vi "TCL Get Signal.vi"(3 "event number":i32, 4 "error in (no error)":errorcluster, 5 "signal name":string, 7 "event file":path) -> (0 "error out":errorcluster, 1 "signal":dbl[](array[numeric]))   [LabVIEW 2010]
doc: "This VI looks up the requested event number and then compares its rf frequency and modulation with the input values. If the event is found, and if the frequency and modulation match, the raw signal of the baseline is returned. Otherwise, an empty array is returned."
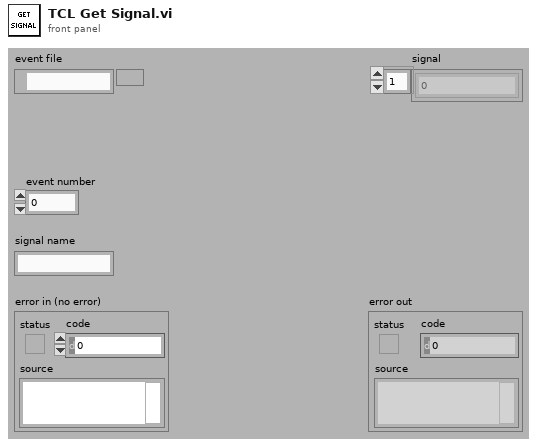
[diagram p1: front panel]
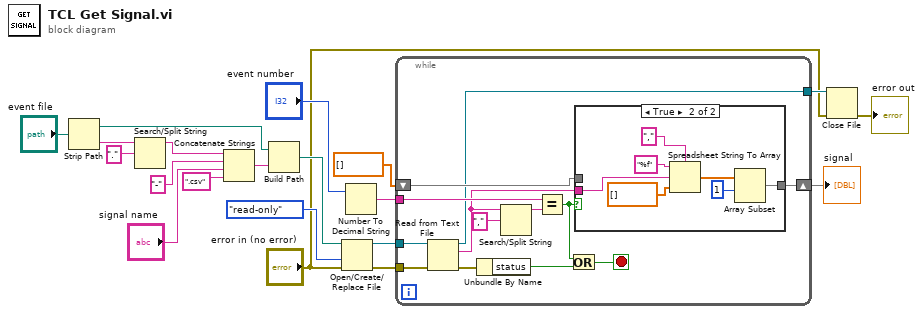
[diagram p0: block diagram]
diagram:
  n1 = Strip Path(path="event file") -> (stripped path=w4:path, name=w3:string)
  n2 = Search/Split String(string=w3, search string/char (-)=".") -> (substring before match=w1:string)  [unwired: 1 in, 2 out]
  n3 = Concatenate Strings(w1, "-" ("string"), "signal name", ".csv" ("string")) -> (w19:string)
  n4 = Build Path(base path=w4, name or relative path=w19) -> (appended path=w16:path)
  n5 = Open/Create/Replace File(file path (use dialog)=w16, error in="error in (no error)", access (0:read/write)=enum16{"read/write", "read-only", "write-only"}."read-only") -> (refnum out=w14:refnum<file>, error out=w13:errorcluster)  [unwired: 3 in, 1 out]
  n6 = Number To Decimal String(number="event number") -> (decimal integer string=w11:string)  [unwired: 1 in]
  n7 = while {
    tunnel: w14 -> [w33]
    tunnel: w13 -> [w32]
    tunnel: w11 -> [w27]
    shift-right: [w24] -> w9
    shift-left: dbl[] [] -> [w25]
    tunnel: [w22] -> w8
    stop <- w30 stop-if-true
    n8 = Read from Text File(file (use dialog)=w33, error in=w32) -> (refnum out=w22:refnum<file>, text=w21:string, error out=w31:errorcluster)  [unwired: 2 in, 1 out]
    n9 = Unbundle By Name(w31) -> ("status"=w29:bool)
    n10 = Search/Split String(string=w21, search string/char (-)=",") -> (substring before match=w23:string)  [unwired: 1 in, 2 out]
    n11 = Equal?(x=w27, y=w23) -> (x = y?=w26:bool)
    n12 = Or(x=w26, y=w29) -> (x .or. y?=w30:bool)
    n13 = case shown="True" w26 {
      tunnel: w25 -> [w34 _]
      tunnel: [w34 w35] -> w24
      tunnel: w21 -> [_ w41]
      frame False {
      }
      frame True {
        n14 = Spreadsheet String To Array(delimiter (Tab)=",", format string="%f", spreadsheet string=w41, array type (2D Dbl)=dbl[] []) -> (array=w36:dbl[])
        n15 = Array Subset(array=w36, index=1) -> (w35:dbl[])  [unwired: 1 in]
      }
    }
  }
  "signal" <- w9
  n16 = Close File(refnum=w8, error in="error in (no error)") -> (error out=→"error out":errorcluster)  [unwired: 1 out]
